vi "Get Data Subset.vi"(8 "error in":errorcluster, 9 "length":i32, 10 "index":i32, 11 "AlicatCommBank in":refnum<class "AlicatCommBank.lvclass">=refnum) -> (0 "error out":errorcluster, 2 "DataOut":refnum<class "Data.lvclass">[](array[class]), 3 "AlicatCommBank out":refnum<class "AlicatCommBank.lvclass">)   [LabVIEW 2014, in "Alicat.lvlib" / "AlicatCommBank.lvclass"]
doc: "Read the data from the individual controllers. This VI will call <B>Translate Data.vi</B> to turn the data into something meaningful. <B>Translate Data.vi</B> is implemented at the child level."
uses:
  AlicatCommBank.lvclass
  Alicat.lvclass
  Data/MC/AlicatMCData.lvclass
  reusable/Data/Data.lvclass
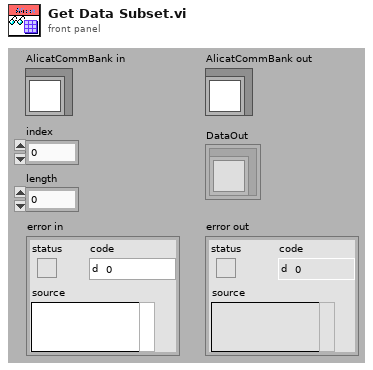
[diagram p1: front panel]
types:
  T1 = cluster{refnum<class "Alicat.lvclass">[], void, void}
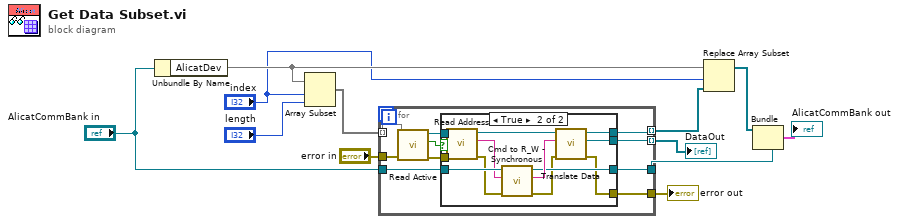
[diagram p0: block diagram]
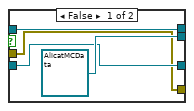
[diagram p2: hidden frame]
diagram:
  n1 = Unbundle By Name("AlicatCommBank in") -> ("AlicatDev"=w4)
  n2 = Array Subset(array=w4, index="index", length="length") -> (w6:void[])
  n3 = for {
    tunnel: w6 -> [w17] mode=indexing
    tunnel: "AlicatCommBank in" -> [w22]
    tunnel: "error in" -> [w16]
    tunnel: [w21] -> w8
    tunnel: [w20] -> w9
    tunnel: [w19] -> w12 mode=indexing
    tunnel: [w18] -> w5 mode=indexing
    n4 = call "Read Active.vi"("error in"=w16, "Alicat in"=w17) -> ("error out"=w14:errorcluster, "Active?"=w13:bool, "Alicat out"=w15:refnum<class "Alicat.lvclass">)  [unwired: 7 in]
    n5 = case shown="True" w13 {
      tunnel: w22 -> [w24 w38]
      tunnel: [w24 w35] -> w21
      tunnel: [w23 w34] -> w20
      tunnel: [refnum<class "AlicatMCData.lvclass"> refnum ("AlicatMData out") w33] -> w19
      tunnel: [w26 w31] -> w18
      tunnel: w15 -> [w26 w28]
      tunnel: w14 -> [w23 w27]
      frame False {
      }
      frame True {
        n6 = call "Read Address.vi"("error in"=w27, "Alicat in"=w28) -> ("error out"=w37:errorcluster, "Address"=w29:string, "Alicat out"=w32:refnum<class "Alicat.lvclass">)  [unwired: 7 in]
        n7 = call-dynamic "Cmd to R_W - Synchronous.vi"("error in"=w37, "write buffer"=w29, "Serial IO in"=w38) -> ("error out"=w30:errorcluster, "read buffer"=w36:string, "Serial IO out"=w35:refnum<class "AlicatCommBank.lvclass">)  [unwired: 6 in]
        n8 = call-dynamic "Translate Data.vi"("error in (no error)"=w30, "BufferIn"=w36, "Alicat in"=w32) -> ("error out"=w34:errorcluster, "DataOut"=w33:refnum<class "Data.lvclass">, "Alicat out"=w31:refnum<class "Alicat.lvclass">)  [unwired: 6 in]
      }
    }
  }
  "error out" <- w9
  "DataOut" <- w12
  n9 = Replace Array Subset(array=w4, new element=w5, index="index") -> (w3:refnum<class "Alicat.lvclass">[])
  n10 = Bundle(cluster=w8, w3) -> (→"AlicatCommBank out":T1)  [unwired: 2 in]
